vi "iRobot UART Write.vi"(8 "error in":errorcluster, 9 "data":u8[](array[numeric]), 11 "UART port in":T1) -> (0 "error out":errorcluster, 3 "UART port out":T1)   [LabVIEW 2010]
doc: "Write data to the UART transmit buffer."
uses:
  UART Port Type.ctl
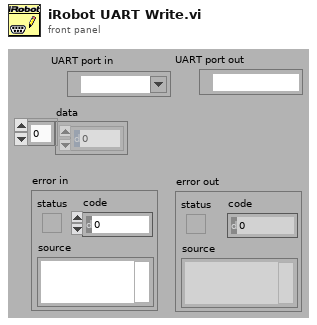
[diagram p1: front panel]
types:
  T1 = typedef "UART Port Type.ctl" = refnum<visa-resource-name>
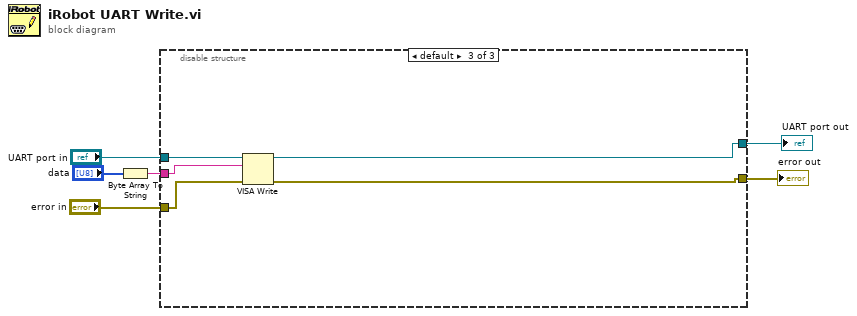
[diagram p0: block diagram]
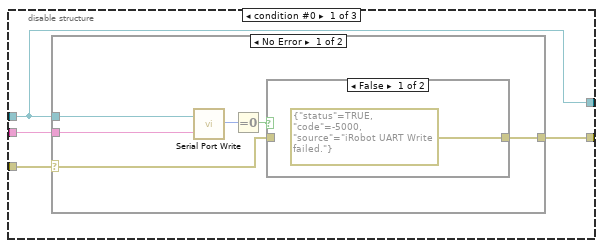
[diagram p2: hidden frame]
diagram:
  n1 = Byte Array To String(unsigned byte array="data") -> (string=w1:string)
  n2 = disable-structure shown="default" {
    disable-tunnel: "UART port in" -> [w7 _ w24]
    disable-tunnel: [w10 _ w20] -> w5
    disable-tunnel: "error in" -> [w9 _ w22]
    disable-tunnel: w1 -> [w8 _ w23]
    disable-tunnel: [w7 _ w21] -> w3
    frame condition #0 {
      n3 = case shown="No Error" w9 {
        selector: w9 -> [w12 w19]
        tunnel: w7 -> [w16 _]
        tunnel: [w13 w19] -> w10
        tunnel: w8 -> [w11 _]
        frame No Error {
          n4 = call <vilib>:"Serial Port Write.vi"("string to write"=w11, "port number"=w16) -> ("error code"=w14:i32)
          n5 = Equal To 0?(x=w14) -> (x = 0?=w15:bool)
          n6 = case shown="False" w15 {
            tunnel: [errorcluster {"status"=TRUE, "code"=-5000, "source"="iRobot UART Write failed."} ("error out") w18] -> w13
            tunnel: w12 -> [_ w18]
            frame False {
            }
            frame True {
              # "No error"
            }
          }
        }
        frame Error {
        }
      }
    }
    frame condition #1 {
      # "To be deployed..."
    }
    frame condition #2 (active) {
      n7 = VISA Write(VISA resource name=w24, write buffer=w23, error in (no error)=w22) -> (VISA resource name out=w21:T1, error out=w20:errorcluster)  [unwired: 1 out]
    }
  }
  "UART port out" <- w3
  "error out" <- w5
